vi "Swerve Wheel.vi"(1 "Wheel":T2(ring)=enum."Front Right", 2 "FeedForward":dbl, 3 "Inputs":dbl[](array[numeric])=[0.0, -0.10193669212665253, -0.14931439584198622, 0.0, 0.0, 10.75, 15.027058927148719, 10.5], 4 "br offset":dbl(knob) scale=-180.0..180.0, 5 "bl offset":dbl(knob) scale=-180.0..180.0, 6 "fr offset":dbl(knob) scale=-180.0..180.0, 7 "fl offset":dbl(knob) scale=-180.0..180.0) -> (0 "Speed":dbl=0.1807923615847232)   [LabVIEW 2019]
uses:
  <vilib>/Rock Robotics/WPI/ThirdParty/Phoenix-LabVIEW/Motor Controller/Controls/CTRE_Phoenix_MotorControl_ControlMode.ctl
  <vilib>/Rock Robotics/Network Tables/NT Write Number.vi
  <vilib>/addons/control/pid/pid.llb/PID (DBL).vi
  <vilib>/addons/control/pid/NI_PID_pid.lvlib
panel:
  out "angle":dbl
  in  "PID gains":T1={"proportional gain (Kc)"=0.009, "integral time (Ti, min)"=0.0, "derivative time (Td, min)"=0.1}
  # "Practice Robot Offsets (3-27-17)\n\nFL:  33\nFR: 32\nBL: 30\nBR:  -178"
  # "Gamer Bot Offsets (3/29/17)\n\nFL: -.7\nFR: -165.5\nBL: 98.2\nBR: -66.7"
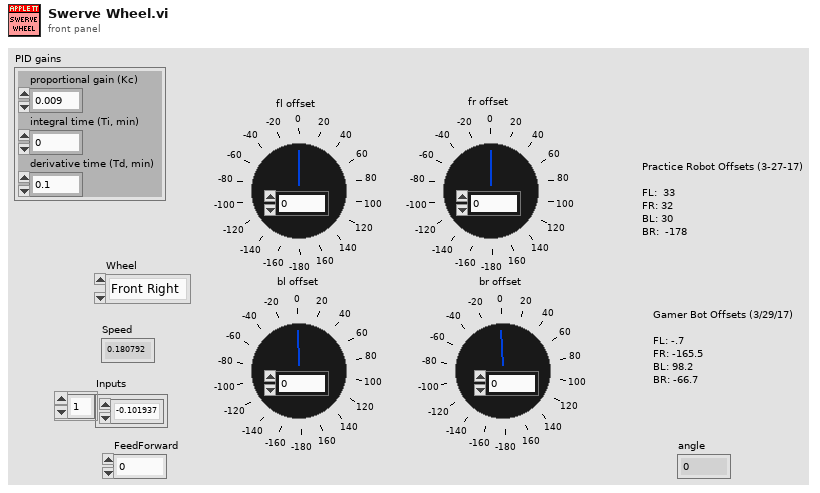
[diagram p1: front panel]
types:
  T1 = cluster{"proportional gain (Kc)":dbl, "integral time (Ti, min)":dbl, "derivative time (Td, min)":dbl}
  T2 = enum16{"Back Left", "Back Right", "Front Left", "Front Right"}
  T3 = typedef "CTRE_Phoenix_MotorControl_ControlMode.ctl" = u16
  T4 = enum16{"Z", "Y", "X", "Rot. Point X", "Rot. Point Y", "Width/2", "Max", "Length/2"}
  T5 = enum16{"Z Axis", "Y", "X", "Rot. Point X", "Rot. Point Y", "Width/2", "Max", "Length/2"}
  T6 = typedef "WPI_MotorControlDeviceRef.ctl" = cluster{"DeviceStatus":errorcluster, "Type":T7, "PWM":cluster{"PWM Channel":T8, "DeadBand":T9}, "CAN":cluster{"Device Number":u8, "SetOutput VI Ref":variant, "GetOutput VI Ref":variant, "Enable VI Ref":variant, "Disable VI Ref":variant, "Data":variant}, "Invert":bool, "DIO PWM":cluster{"PWM \"Enable\" Channel":T8, "DIOChannel":T10, "PWM Rate":dbl}}
  T7 = typedef "WPI_MotorControlType.ctl" = enum16{"PWM", "CAN", "DIO PWM"}
  T8 = typedef "FPGA_DIOPWMChannel.ctl" = enum8{"PWM 0", "PWM 1", "PWM 2", "PWM 3", "PWM 4", "PWM 5", "PWM 6", "PWM 7", "PWM 8", "PWM 9", "PWM MXP 0", "PWM MXP 1", "PWM MXP 2", "PWM MXP 3", "PWM MXP 4", "PWM MXP 5", "PWM MXP 6", "PWM MXP 7", "PWM MXP 8", "PWM MXP 9", "Invalid"}
  T9 = typedef "WPI_PWMDeadband.ctl" = cluster{"Name":string, "maxPositivePwm":i32, "minPositivePwm":i32, "centerPwm":i32, "maxNegativePwm":i32, "minNegativePwm":i32, "angularRange":u16}
  T10 = typedef "FPGA_DIOChannel.ctl" = enum8{"DIO 0", "DIO 1", "DIO 2", "DIO 3", "DIO 4", "DIO 5", "DIO 6", "DIO 7", "DIO 8", "DIO 9", "DIO MXP 0", "DIO MXP 1", "DIO MXP 2", "DIO MXP 3", "DIO MXP 4", "DIO MXP 5", "DIO MXP 6", "DIO MXP 7", "DIO MXP 8", "DIO MXP 9", "DIO MXP 10", "DIO MXP 11", "DIO MXP 12", "DIO MXP 13", "DIO MXP 14", "DIO MXP 15", "SPI Port CS1", "SPI Port CS2", "SPI Port CS3", "SPI Port MISO", "SPI Port MOSI", "Invalid"}
  T11 = typedef "WPI_PotentiometerDevRef.ctl" = cluster{"DevStatus":errorcluster, "Analog Channel":T12, "Invert Output":bool}
  T12 = typedef "FPGA_AIChannel.ctl" = enum8{"AI 0", "AI 1", "AI 2", "AI 3", "AI MXP 0", "AI MXP 1", "AI MXP 2", "AI MXP 3", "Invalid"}
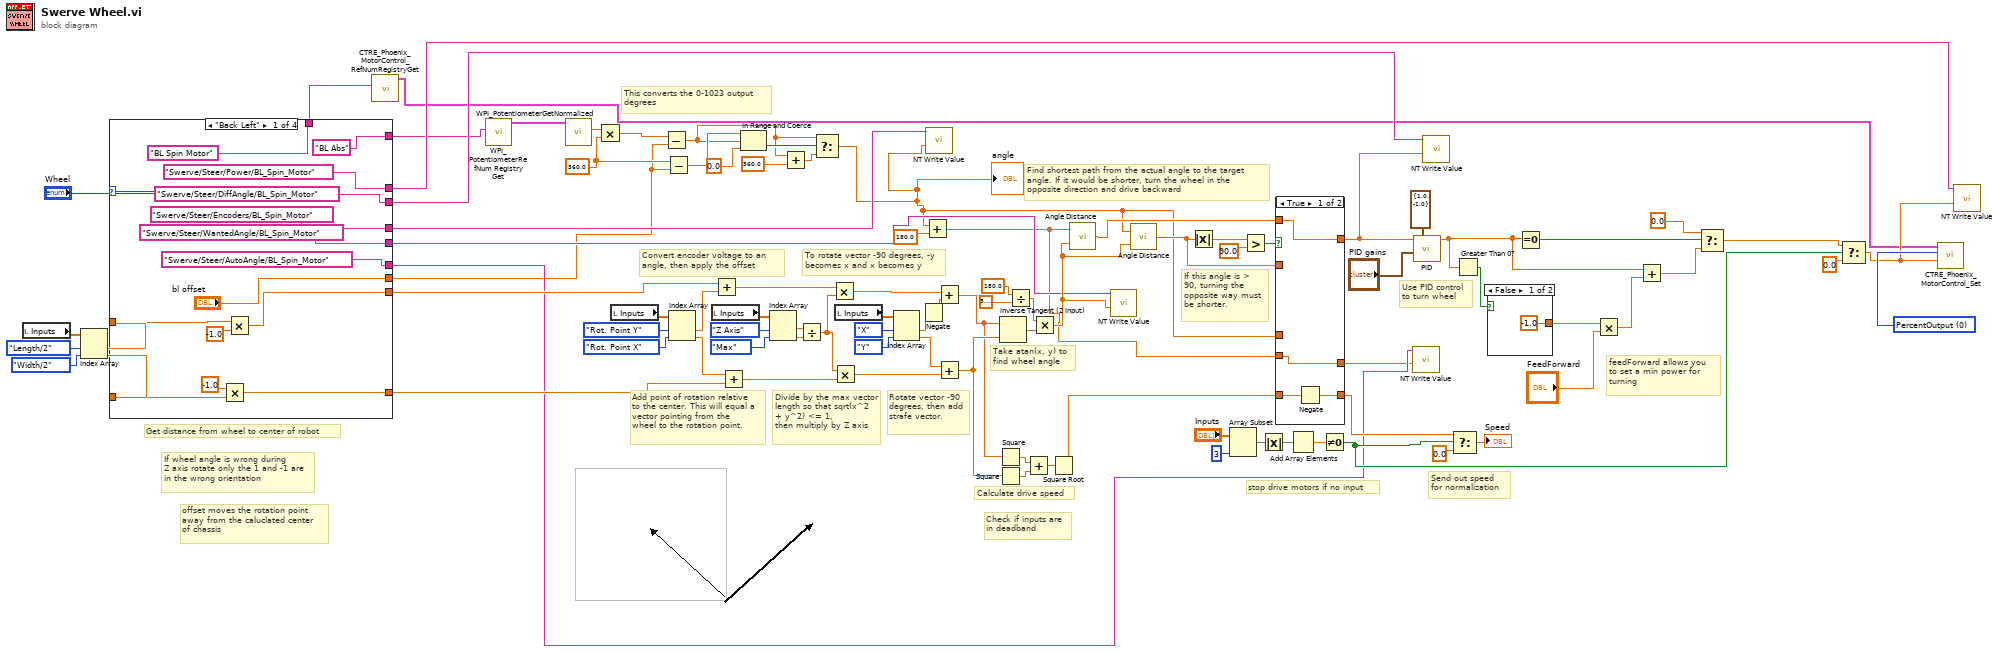
[diagram p0: block diagram]
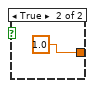
[diagram p2: hidden frame]
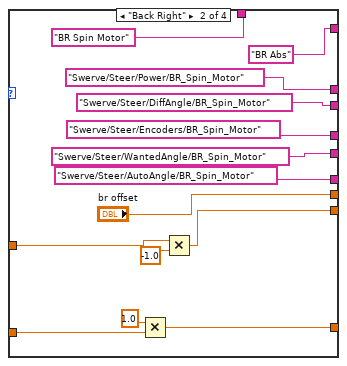
[diagram p4: hidden frame]
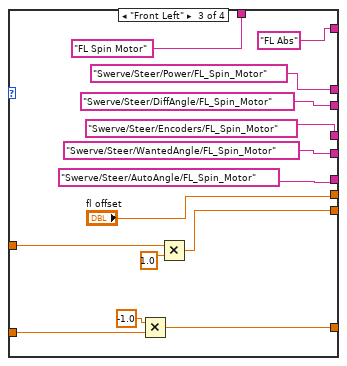
[diagram p5: hidden frame]
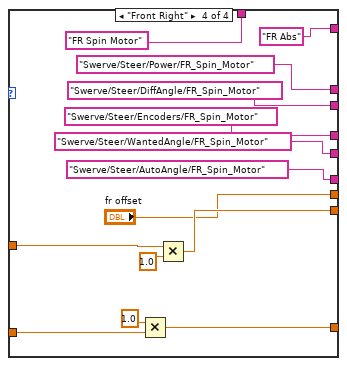
[diagram p6: hidden frame]
diagram:
  w37 = T3 0 items=["PercentOutput"=0, "Position"=1, "Velocity"=2, "Current"=3, "Follower"=5, "MotionProfile"=6, "MotionMagic"=7, "MotionMagicArc"=8, "MotionProfileArc"=10, "Disabled"=15] ("Control Mode")
  w3 = 360.0
  # "feedForward allows you \nto set a min power for \nturning"
  # "stop drive motors if no input"
  # "This converts the 0-1023 output \ndegrees"
  # "offset moves the rotation point\naway from the caluclated center\nof chassis"
  # "If wheel angle is wrong during\nZ axis rotate only the 1 and -1 are\nin the wrong orientation"
  # "To rotate vector -90 degrees, -y becomes x and x becomes y"
  # "Divide by the max vector length so that sqrt(x^2 + y^2) <= 1,\nthen multiply by Z axis"
  # "Add point of rotation relative to the center. This will equal a vector pointing from the\nwheel to the rotation point."
  # "Send out speed\nfor normalization"
  # "Check if inputs are\nin deadband"
  # "Convert encoder voltage to an angle, then apply the offset"
  # "If this angle is > 90, turning the opposite way must be shorter."
  # "Use PID control\nto turn wheel"
  # "Find shortest path from the actual angle to the target angle. If it would be shorter, turn the wheel in the opposite direction and drive backward"
  # "Take atan(x, y) to find wheel angle"
  # "Calculate drive speed"
  # "Rotate vector -90 degrees, then add strafe vector."
  # "Get distance from wheel to center of robot"
  n1 = local read "Inputs"() -> (w49:dbl[])
  n2 = Index Array(array=w49, index #1=T4."Length/2", index #2=T4."Width/2") -> (element #1=w47:dbl, element #2=w46:dbl)
  n3 = case shown="\"Back Left\"" "Wheel" {
    tunnel: ["BL Spin Motor" "BR Spin Motor" "FL Spin Motor" "FR Spin Motor"] -> w14
    tunnel: ["bl offset" "br offset" "fl offset" "fr offset"] -> w1
    tunnel: w47 -> [w104 w118 w132 w146]
    tunnel: w46 -> [w102 w116 w131 w144]
    tunnel: [w101 w115 w130 w143] -> w71
    tunnel: [w100 w114 w129 w142] -> w67
    tunnel: ["Swerve/Steer/Encoders/BL_Spin_Motor" "Swerve/Steer/Encoders/BR_Spin_Motor" "Swerve/Steer/Encoders/FL_Spin_Motor" "Swerve/Steer/Encoders/FR_Spin_Motor"] -> w35
    tunnel: ["Swerve/Steer/WantedAngle/BL_Spin_Motor" "Swerve/Steer/WantedAngle/BR_Spin_Motor" "Swerve/Steer/WantedAngle/FL_Spin_Motor" "Swerve/Steer/WantedAngle/FR_Spin_Motor"] -> w33
    tunnel: ["Swerve/Steer/DiffAngle/BL_Spin_Motor" "Swerve/Steer/DiffAngle/BR_Spin_Motor" "Swerve/Steer/DiffAngle/FL_Spin_Motor" "Swerve/Steer/DiffAngle/FR_Spin_Motor"] -> w32
    tunnel: ["Swerve/Steer/Power/BL_Spin_Motor" "Swerve/Steer/Power/BR_Spin_Motor" "Swerve/Steer/Power/FL_Spin_Motor" "Swerve/Steer/Power/FR_Spin_Motor"] -> w30
    tunnel: ["Swerve/Steer/AutoAngle/BL_Spin_Motor" "Swerve/Steer/AutoAngle/BR_Spin_Motor" "Swerve/Steer/AutoAngle/FL_Spin_Motor" "Swerve/Steer/AutoAngle/FR_Spin_Motor"] -> w17
    tunnel: ["BL Abs" ("refnum name") "BR Abs" ("refnum name") "FL Abs" ("refnum name") "FR Abs" ("refnum name")] -> w12
    frame "Back Left" {
      n4 = Multiply(x=-1.0 ("y"), y=w102) -> (x*y=w100:dbl)
      n5 = Multiply(x=w104, y=-1.0) -> (x*y=w101:dbl)
    }
    frame "Back Right" {
      n6 = Multiply(x=1.0 ("y"), y=w116) -> (x*y=w114:dbl)
      n7 = Multiply(x=w118, y=-1.0) -> (x*y=w115:dbl)
    }
    frame "Front Left" {
      n8 = Multiply(x=-1.0 ("y"), y=w131) -> (x*y=w129:dbl)
      n9 = Multiply(x=w132, y=1.0) -> (x*y=w130:dbl)
    }
    frame "Front Right" {
      n10 = Multiply(x=1.0 ("y"), y=w144) -> (x*y=w142:dbl)
      n11 = Multiply(x=w146, y=1.0) -> (x*y=w143:dbl)
    }
  }
  n12 = call <vilib>:"CTRE_Phoenix_MotorControl_RefNumRegistryGet.vi"("refnum name"=w14) -> ("PhoenixMotorControlDevRef"=w13:T6)  [unwired: 9 in, 1 out]
  n13 = call <vilib>:"WPI_PotentiometerRefNum Registry Get.vi"("refnum name"=w12) -> ("PotDevRef"=w40:T11)  [unwired: 9 in, 1 out]
  n14 = call <vilib>:"WPI_PotentiometerGetNormalized.vi"("PotDevRef"=w40) -> ("Normalized Value"=w11:dbl)  [unwired: 8 in, 2 out]
  n15 = Multiply(x=w11, y=w3) -> (x*y=w4:dbl)
  n16 = local read "Inputs"() -> (w69:dbl[])
  n17 = Subtract(x=w4, y=w1) -> (x-y=w5:dbl)
  n18 = Subtract(x=w3, y=w1) -> (x-y=w10:dbl)
  n19 = Index Array(array=w69, index #1=T4."Rot. Point Y", index #2=T4."Rot. Point X") -> (element #1=w65:dbl, element #2=w66:dbl)
  n20 = local read "Inputs"() -> (w63:dbl[])
  n21 = Add(x=w71, y=w65) -> (x+y=w45:dbl)
  n22 = Add(x=w66, y=w67) -> (x+y=w59:dbl)
  n23 = In Range and Coerce(upper limit=w10, x=w5, lower limit=0.0) -> (In Range?=w8:bool)  [unwired: 1 out]
  n24 = Index Array(array=w63, index #1=T5."Z Axis", index #2=T4."Max") -> (element #1=w60:dbl, element #2=w61:dbl)
  n25 = Add(x=w5, y=360.0) -> (x+y=w7:dbl)
  n26 = Divide(x=w60, y=w61) -> (x/y=w36:dbl)
  n27 = Select(t=w5, s=w8, f=w7) -> (s? t:f=w2:dbl)
  "angle" <- w2
  n28 = Multiply(x=w45, y=w36) -> (x*y=w43:dbl)
  n29 = Multiply(x=w36, y=w59) -> (x*y=w54:dbl)
  n30 = local read "Inputs"() -> (w57:dbl[])
  n31 = Index Array(array=w57, index #1=T4."X", index #2=T4."Y") -> (element #1=w41:dbl, element #2=w53:dbl)
  n32 = Negate(x=w41) -> (-x=w42:dbl)
  n33 = Add(x=w2, y=180.0 ("f")) -> (x+y=w16:dbl)
  n34 = call-poly <vilib>:"NT Write Value.vi"("Numeric"=w2, "Name"=w35) -> ()  [unwired: 9 in, 1 out]
  n35 = Add(x=w43, y=w42) -> (x+y=w51:dbl)
  n36 = Add(x=w53, y=w54) -> (x+y=w52:dbl)
  n37 = Square(x=w51) -> (x^2=w55:dbl)
  n38 = Square(x=w52) -> (x^2=w88:dbl)
  n39 = Inverse Tangent (2 Input)(1:w52, 2:w51) -> (0:w89:dbl)
  n40 = Divide(x=180.0 ("y"), y=3.141592653589793) -> (x/y=w86:dbl)
  n41 = Add(x=w55, y=w88) -> (x+y=w87:dbl)
  n42 = Multiply(x=w86, y=w89) -> (x*y=w34:dbl)
  n43 = Square Root(x=w87) -> (sqrt(x)=w80:dbl)
  n44 = call "Angle Distance.vi"("target angle"=w34, "current angle"=w16) -> ("distance"=w38:dbl)
  n45 = call-poly <vilib>:"NT Write Value.vi"("Numeric"=w34, "Name"=w33) -> ()  [unwired: 9 in, 1 out]
  n46 = call "Angle Distance.vi"("target angle"=w34, "current angle"=w2) -> ("distance"=w39:dbl)
  n47 = Absolute Value(x=w39) -> (abs(x)=w81:dbl)
  n48 = Array Subset(array="Inputs", length=3) -> (w76:dbl[])  [unwired: 1 in]
  n49 = Greater?(x=w81, y=90.0) -> (0:w18:bool)
  n50 = Absolute Value(x=w76) -> (abs(x)=w72:dbl[])
  n51 = case shown="True" w18 {
    tunnel: w38 -> [w150 _]
    tunnel: w39 -> [_ w155]
    tunnel: [w151 w154] -> w75
    tunnel: w80 -> [w152 w154]
    tunnel: [w150 w155] -> w20
    tunnel: w2 -> [_ w153]
    tunnel: w16 -> [w149 _]
    tunnel: [w149 w153] -> w15
    frame True {
      n52 = Negate(x=w152) -> (-x=w151:dbl)
    }
    frame False {
    }
  }
  n53 = Add Array Elements(numeric array=w72) -> (sum=w90:dbl)
  n54 = Not Equal To 0?(x=w90) -> (x != 0?=w19:bool)
  n55 = call-poly <vilib>:"NT Write Value.vi"("Numeric"=w15, "Name"=w17) -> ()  [unwired: 9 in, 1 out]
  n56 = call-poly <vilib>:"PID.vi"("output range"=cluster{"output high":dbl, "output low":dbl} {"output high"=1.0, "output low"=-1.0}, "PID gains"="PID gains", "setpoint"=w20) -> ("output"=w23:dbl)  [unwired: 7 in, 1 out]
  n57 = call-poly <vilib>:"NT Write Value.vi"("Numeric"=w20, "Name"=w32) -> ()  [unwired: 9 in, 1 out]
  n58 = Select(t=w75, s=w19, f=0.0) -> (s? t:f=→"Speed":dbl)
  n59 = Greater Than 0?(x=w23) -> (x > 0?=w22:bool)
  n60 = case shown="False" w22 {
    tunnel: [-1.0 ("x") 1.0 ("x")] -> w21
    frame False {
    }
    frame True {
    }
  }
  n61 = Equal To 0?(x=w23) -> (x = 0?=w29:bool)
  n62 = Multiply(x=w21, y="FeedForward") -> (x*y=w24:dbl)
  n63 = Add(x=w23, y=w24) -> (x+y=w26:dbl)
  n64 = Select(t=0.0, s=w29, f=w26) -> (s? t:f=w27:dbl)
  n65 = Select(t=w27, s=w19, f=0.0) -> (s? t:f=w31:dbl)
  n66 = call <vilib>:"CTRE_Phoenix_MotorControl_Set.vi"("Output"=w31, "Control Mode"=w37, "PhoenixMotorControlDevRef"=w13) -> ()  [unwired: 7 in, 2 out]
  n67 = call-poly <vilib>:"NT Write Value.vi"("Numeric"=w31, "Name"=w30) -> ()  [unwired: 9 in, 1 out]
